vi "Init.vi"(8 "error in (no error)":errorcluster, 10 "EnQr":refnum<class "Message Enqueuer.lvclass">) -> (0 "error out":errorcluster, 3 "Event API out":refnum<class "EventAPI.lvclass">)   [LabVIEW 2020, in "Volatus.lvlib" / "EventAPI.lvclass"]
uses:
  EventAPI.lvclass
  <vilib>/ActorFramework/Message Enqueuer/Message Enqueuer.lvclass
  EventAPI.lvclass/EventAPI.ctl
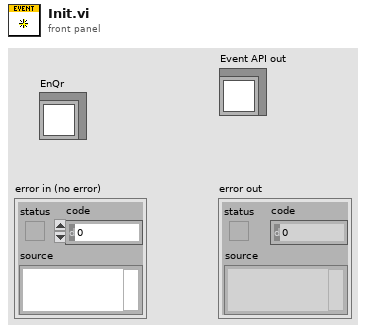
[diagram p1: front panel]
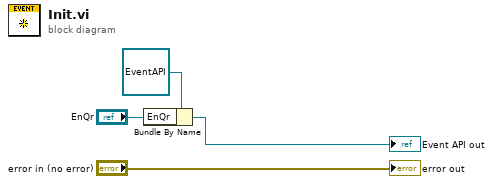
[diagram p0: block diagram]
diagram:
  n1 = Bundle By Name(cluster=refnum<class "EventAPI.lvclass"> refnum ("Event API in"), "EnQr"="EnQr") -> (→"Event API out":refnum<class "EventAPI.lvclass">)
  "error out" <- "error in (no error)"
